vi "lock.vi"(6 "timeout (2000ms)":i32=2000, 8 "error in (no error)":errorcluster, 11 "Client in":refnum<class "Client.lvclass">) -> (0 "error out":errorcluster, 1 "timed out":bool, 3 "Client out":refnum<class "Client.lvclass">, 4 "remaining (ms)":i32=2000, 5 "locked":bool)   [LabVIEW 2013, in "MQTT Client.lvlib" / "Client.lvclass"]
uses:
  Client.lvclass
  Client.lvclass/Client.ctl
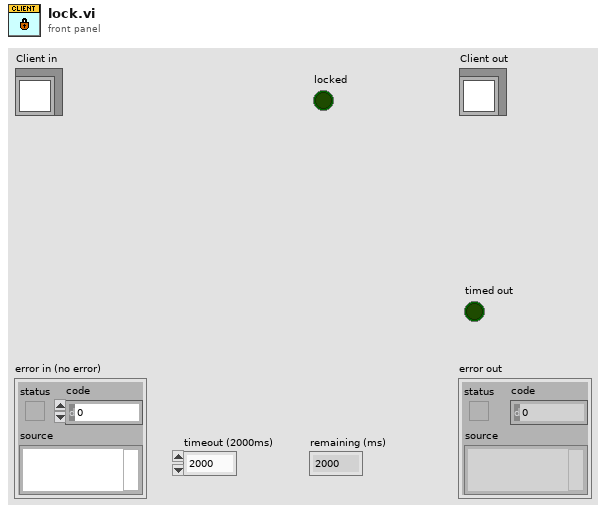
[diagram p1: front panel]
types:
  T1 = typedef "Semaphore RefNum" = refnum<k1>
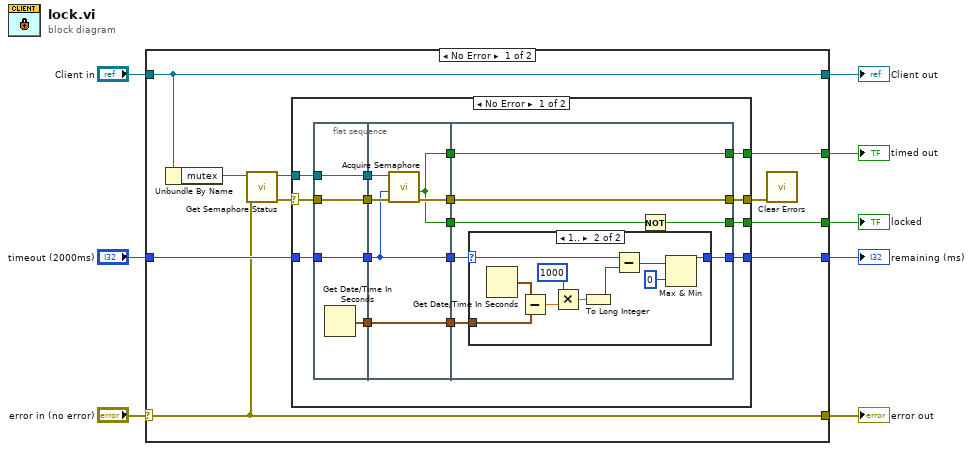
[diagram p0: block diagram]
diagram:
  n1 = case shown="No Error" "error in (no error)" {
    selector: "error in (no error)" -> [w10 w67]
    tunnel: [w10 w67] -> w7
    tunnel: [w12 w66] -> w5
    tunnel: "Client in" -> [w12 w66]
    tunnel: "timeout (2000ms)" -> [w15 w65]
    tunnel: [w13 _] -> w3
    tunnel: [w11 w65] -> w2
    tunnel: [w9 _] -> w1
    frame No Error {
      n2 = Unbundle By Name(w12) -> ("mutex"=w18:T1)
      n3 = call <vilib>:"Get Semaphore Status.vi"("error in (no error)"=w10, "semaphore"=w18) -> ("error out"=w17:errorcluster, "semaphore out"=w16:T1)  [unwired: 4 in, 4 out]
      n4 = case shown="No Error" w17 {
        selector: w17 -> [w33 w64]
        tunnel: w16 -> [w34 _]
        tunnel: w15 -> [w32 w63]
        tunnel: [w31 w64] -> w14
        tunnel: [w30 _] -> w13
        tunnel: [w21 w63] -> w11
        tunnel: [w19 _] -> w9
        frame No Error {
          n5 = flat-sequence {
            tunnel: w32 -> [w36]
            tunnel: w33 -> [w37]
            tunnel: w34 -> [w38]
            tunnel: [w38] -> w27
            tunnel: [w37] -> w26
            tunnel: [w36] -> w25
            tunnel: [w35] -> w24
            tunnel: [w42] -> w29
            tunnel: [w39] -> w28
            tunnel: w27 -> [w44]
            tunnel: w26 -> [w43]
            tunnel: w25 -> [w40]
            tunnel: w24 -> [w41]
            tunnel: [w41] -> w23
            tunnel: [w40] -> w22
            tunnel: [w39] -> w20
            tunnel: [w46] -> w30
            tunnel: [w51] -> w31
            tunnel: w29 -> [w51]
            tunnel: w28 -> [w50]
            tunnel: w23 -> [w49]
            tunnel: w22 -> [w47]
            tunnel: [w48] -> w21
            tunnel: w20 -> [w45]
            tunnel: [w45] -> w19
            frame #0 {
              n6 = Get Date/Time In Seconds() -> (seconds since 1Jan1904=w35:timestamp)
            }
            frame #1 {
              n7 = call <vilib>:"Acquire Semaphore.vi"("error in (no error)"=w43, "ms timeout (-1)"=w40, "semaphore"=w44) -> ("error out"=w42:errorcluster, "timed out"=w39:bool)  [unwired: 2 in, 1 out]
            }
            frame #2 {
              n8 = case shown="1.." w47 {
                selector: w47 -> [w52 w53]
                tunnel: w49 -> [_ w62]
                tunnel: [w52 w54] -> w48
                frame Default {
                }
                frame 1.. {
                  n9 = Get Date/Time In Seconds() -> (seconds since 1Jan1904=w61:timestamp)
                  n10 = Subtract(x=w61, y=w62) -> (x-y=w60:dbl)
                  n11 = Multiply(x=1000 ("timeout (2000ms)"), y=w60) -> (x*y=w58:dbl)
                  n12 = To Long Integer(number=w58) -> (32bit integer=w57:i32)
                  n13 = Subtract(x=w53, y=w57) -> (x-y=w56:i32)
                  n14 = Max & Min(x=w56, y=0) -> (max(x,y)=w54:i32)  [unwired: 1 out]
                }
              }
              n15 = Not(x=w50) -> (.not. x?=w46:bool)
            }
          }
        }
        frame Error {
        }
      }
      n16 = call <vilib>:"Clear Errors.vi"("error in (no error)"=w14) -> ()  [unwired: 6 in, 1 out]
    }
    frame Error {
    }
  }
  "error out" <- w7
  "Client out" <- w5
  "locked" <- w3
  "remaining (ms)" <- w2
  "timed out" <- w1
